vi "Example virtual calibration data generator.vi"(0 "t0_U_cal t0 (m/s)":dbl[](array[numeric])=[0.0018065055399, 0.51984069575, 0.9737, 2.0137147675, 3.036660399, 4.008390834, 5.0589598065, 6.0604802741, 7.0995183408, 8.0765049797, 9.0912586991, 10.081448823, 11.876663392], 1 "t0_Vout_cal t0 (V)":dbl[](array[numeric])=[0.053989069621, 0.62774937057, 0.93949993515, 1.4010595347, 1.714702877, 1.9456688245, 2.1571508535, 2.3284715843, 2.4859547348, 2.6192157707, 2.7474417318, 2.8639088415, 3.0588901316], 3 "time fraction (0...1)":dbl=0.5 min=0.0 max=1.0, 5 "t0_Ta_cal (°C)":dbl[](array[numeric])=[20.994930577, 20.998488576, 21.001202392, 21.00530951, 21.005031565, 21.012907585, 21.024551146, 21.046328275, 21.072132623, 21.111764011, 21.153745433, 21.182721788, 21.208832231], 7 "t1_Vout_cal t0 (V)":dbl[](array[numeric])=[0.045499523163, 0.60666541417, 0.91558652878, 1.3778238233, 1.6925483742, 1.9226294759, 2.1202740657, 2.2916270447, 2.4508691012, 2.5910185776, 2.7221374766, 2.8443260727, 3.0437243334], 9 "t1_U_cal t0 (m/s)":dbl[](array[numeric])=[0.021020600342, 0.51776852003, 0.98012050062, 2.0073197538, 3.0227502489, 3.9782177479, 4.9506397512, 5.9384973419, 6.9603671247, 7.9606730411, 8.9790875099, 10.010118367, 11.844900957], 11 "t1_Ta_cal (°C)":dbl[](array[numeric])=[21.415303275, 21.38340196, 21.380579107, 21.375484666, 21.374167855, 21.37609939, 21.376411452, 21.399550636, 21.436538733, 21.478179347, 21.519214886, 21.536252007, 21.540514259], 12 "Overheat ratio":dbl=1.7, 13 "Gain":dbl=10.0, 14 "Offset (V)":dbl=0.512) -> (4 "t_frac Calibration data":T1={"X cal.[]"=[0.16942387073906073, 0.3571463864829161, 0.4649272045522078, 0.6384095030771939, 0.7632235157537435, 0.8589678745414981, 0.9489717058438498, 1.0240141417905662, 1.0951488178464426, 1.1566490826880553, 1.2166980237427845, 1.2717330176412438, 1.3654642977024674], "Re cal.[]"=[0.0003549732812892601, 0.10214643281768965, 0.19132665434147333, 0.39568017737456973, 0.5966818576867157, 0.7876060754864341, 0.9940059313339666, 1.190731239913453, 1.3947958933586706, 1.5865981769860278, 1.7857758481557438, 1.9801490739357872, 2.332620901742986], "a1[]"=[0.5422442754565113, 0.6848331445720253, 1.0026861494680874, 1.394179926934208, 1.8022568311200722, 2.1436691011118443, 2.4573774667113204, 2.7451146877065913, 2.9937157196852064, 3.217822590174205, 3.424366908750728, 3.6461309534080004], "a2[]"=[-0.7595725454163121, 1.0197881628604482, 0.7741344852897616, 1.927764485021313, 2.4453609640659906, 1.4997878970452068, 2.727694680301364, 1.7175948982636757, 2.4538859657545333, 1.511346978354529, 1.8273792682683536, 2.4393015310094333], "a3[]"=[4.046251683803012, 2.8127827457089394, 1.361156267749989, -1.5651263013416128, -4.612450848415237, 1.7996431474362735, -7.200648409580028, 0.2793016807904881, -6.849691205223936, 2.314255218633881, 2.2697753416122333, -13.012206434266801]}, 10 "t0 Calibration data":T1={"X cal.[]"=[0.16942387073906073, 0.3571463864829161, 0.4649272045522078, 0.6384095030771939, 0.7632235157537435, 0.8589678745414981, 0.9489717058438498, 1.0240141417905662, 1.0951488178464426, 1.1566490826880553, 1.2166980237427845, 1.2717330176412438, 1.3654642977024674], "Re cal.[]"=[0.0003549732812892601, 0.10214643281768965, 0.19132665434147333, 0.39568017737456973, 0.5966818576867157, 0.7876060754864341, 0.9940059313339666, 1.190731239913453, 1.3947958933586706, 1.5865981769860278, 1.7857758481557438, 1.9801490739357872, 2.332620901742986], "a1[]"=[0.5422442754565113, 0.6848331445720253, 1.0026861494680874, 1.394179926934208, 1.8022568311200722, 2.1436691011118443, 2.4573774667113204, 2.7451146877065913, 2.9937157196852064, 3.217822590174205, 3.424366908750728, 3.6461309534080004], "a2[]"=[-0.7595725454163121, 1.0197881628604482, 0.7741344852897616, 1.927764485021313, 2.4453609640659906, 1.4997878970452068, 2.727694680301364, 1.7175948982636757, 2.4538859657545333, 1.511346978354529, 1.8273792682683536, 2.4393015310094333], "a3[]"=[4.046251683803012, 2.8127827457089394, 1.361156267749989, -1.5651263013416128, -4.612450848415237, 1.7996431474362735, -7.200648409580028, 0.2793016807904881, -6.849691205223936, 2.314255218633881, 2.2697753416122333, -13.012206434266801]}, 15 "t1* Calibration data":T1={"X cal.[]"=[0.16942387073906073, 0.3571463864829161, 0.4649272045522078, 0.6384095030771939, 0.7632235157537435, 0.8589678745414981, 0.9489717058438498, 1.0240141417905662, 1.0951488178464426, 1.1566490826880553, 1.2166980237427845, 1.2717330176412438, 1.3654642977024674], "Re cal.[]"=[0.0003549732812892601, 0.10214643281768965, 0.19132665434147333, 0.39568017737456973, 0.5966818576867157, 0.7876060754864341, 0.9940059313339666, 1.190731239913453, 1.3947958933586706, 1.5865981769860278, 1.7857758481557438, 1.9801490739357872, 2.332620901742986], "a1[]"=[0.5422442754565113, 0.6848331445720253, 1.0026861494680874, 1.394179926934208, 1.8022568311200722, 2.1436691011118443, 2.4573774667113204, 2.7451146877065913, 2.9937157196852064, 3.217822590174205, 3.424366908750728, 3.6461309534080004], "a2[]"=[-0.7595725454163121, 1.0197881628604482, 0.7741344852897616, 1.927764485021313, 2.4453609640659906, 1.4997878970452068, 2.727694680301364, 1.7175948982636757, 2.4538859657545333, 1.511346978354529, 1.8273792682683536, 2.4393015310094333], "a3[]"=[4.046251683803012, 2.8127827457089394, 1.361156267749989, -1.5651263013416128, -4.612450848415237, 1.7996431474362735, -7.200648409580028, 0.2793016807904881, -6.849691205223936, 2.314255218633881, 2.2697753416122333, -13.012206434266801]})   [LabVIEW 2022 SP3]
doc: "Example VI for how to pre-process and make use of two sequential calibration datasets to generate a virtual calibration at some fractional time between the two calibration datasets.\nPN 15-OCT-24."
uses:
  Ctls/Calibration data.ctl
panel:
  out "Calibration curves":cluster{dbl[], dbl[]}[](graph)=[{[0.17351078077836318, 0.35960238349240253, 0.46891791081947753, 0.6413681992780179, 0.7657591156025723, 0.8611448971603233, 0.951297198203673, 1.0263676092211313, 1.0969658195169174, 1.1579995632331852, 1.2177718423536772, 1.2728558335390798, 1.3667235881026694], [0.0003549732812892601, 0.10214643281768965, 0.19132665434147333, 0.39568017737456973, 0.5966818576867157, 0.7876060754864341, 0.9940059313339666, 1.190731239913453, 1.3947958933586706, 1.5865981769860278, 1.7857758481557438, 1.9801490739357872, 2.332620901742986]}, {[0.16533696069975826, 0.3546903894734296, 0.4609364982849381, 0.6354508068763699, 0.7606879159049147, 0.856790851922673, 0.9466462134840266, 1.0216606743600007, 1.0933318161759675, 1.1552986021429255, 1.2156242051318917, 1.2706102017434078, 1.3642050073022656], [0.0003549732812892601, 0.10214643281768965, 0.19132665434147333, 0.39568017737456973, 0.5966818576867157, 0.7876060754864341, 0.9940059313339666, 1.190731239913453, 1.3947958933586706, 1.5865981769860278, 1.7857758481557438, 1.9801490739357872, 2.332620901742986]}, {[0.16942387073906073, 0.3571463864829161, 0.4649272045522078, 0.6384095030771939, 0.7632235157537435, 0.8589678745414981, 0.9489717058438498, 1.0240141417905662, 1.0951488178464426, 1.1566490826880553, 1.2166980237427845, 1.2717330176412438, 1.3654642977024674], [0.0003549732812892601, 0.10214643281768965, 0.19132665434147333, 0.39568017737456973, 0.5966818576867157, 0.7876060754864341, 0.9940059313339666, 1.190731239913453, 1.3947958933586706, 1.5865981769860278, 1.7857758481557438, 1.9801490739357872, 2.332620901742986]}]
  # "Note: t0 and t1 arrays must have the same length."
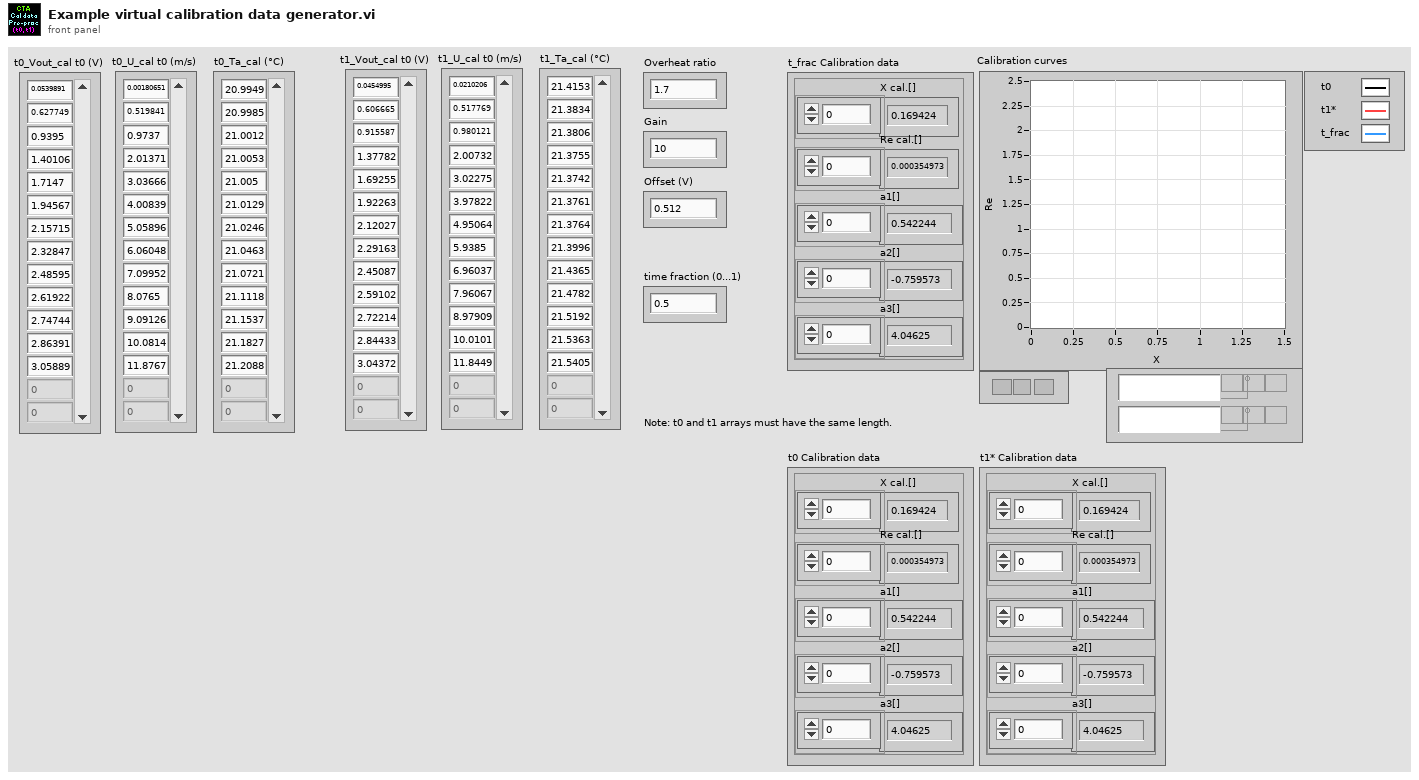
[diagram p1: front panel]
types:
  T1 = typedef "Calibration data.ctl" = cluster{"X cal.[]":dbl[], "Re cal.[]":dbl[], "a1[]":dbl[], "a2[]":dbl[], "a3[]":dbl[]}
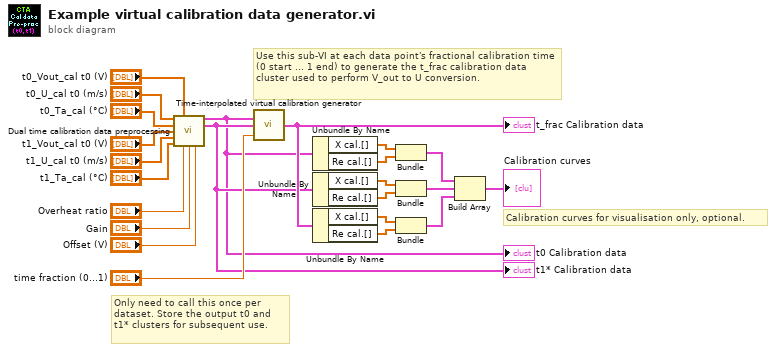
[diagram p0: block diagram]
diagram:
  # "Calibration curves for visualisation only, optional."
  # "Use this sub-VI at each data point's fractional calibration time (0 start ... 1 end) to generate the t_frac calibration data cluster used to perform V_out to U conversion."
  # "Only need to call this once per dataset. Store the output t0 and t1* clusters for subsequent use."
  n1 = call "Dual time calibration data preprocessing.vi"("t0_U_cal t0 (m/s)"="t0_U_cal t0 (m/s)", "t0_Vout_cal t0 (V)"="t0_Vout_cal t0 (V)", "t0_Ta_cal (°C)"="t0_Ta_cal (°C)", "t1_Vout_cal t0 (V)"="t1_Vout_cal t0 (V)", "t1_U_cal t0 (m/s)"="t1_U_cal t0 (m/s)", "t1_Ta_cal (°C)"="t1_Ta_cal (°C)", "Overheat ratio"="Overheat ratio", "Gain"="Gain", "Offset (V)"="Offset (V)") -> ("t0 Calibration data"=w1:T1, "t1* Calibration data"=w2:T1)  [unwired: 5 in]
  "t0 Calibration data" <- w1
  "t1* Calibration data" <- w2
  n2 = call "Time-interpolated virtual calibration generator.vi"("time fraction (0...1)"="time fraction (0...1)", "t1* Calibration data"=w2, "t0 Calibration data"=w1) -> ("t_frac Calibration data"=w3:T1)
  "t_frac Calibration data" <- w3
  n3 = Unbundle By Name(w1) -> ("X cal.[]"=w9:dbl[], "Re cal.[]"=w6:dbl[])
  n4 = Unbundle By Name(w2) -> ("X cal.[]"=w8:dbl[], "Re cal.[]"=w5:dbl[])
  n5 = Unbundle By Name(w3) -> ("X cal.[]"=w7:dbl[], "Re cal.[]"=w4:dbl[])
  n6 = Bundle("X cal.[]"=w9, "Re cal.[]"=w6) -> (w11:cluster{"X cal.[]":dbl[], "Re cal.[]":dbl[]})  [unwired: 1 in]
  n7 = Bundle("X cal.[]"=w8, "Re cal.[]"=w5) -> (w12:cluster{"X cal.[]":dbl[], "Re cal.[]":dbl[]})  [unwired: 1 in]
  n8 = Bundle("X cal.[]"=w7, "Re cal.[]"=w4) -> (w13:cluster{"X cal.[]":dbl[], "Re cal.[]":dbl[]})  [unwired: 1 in]
  n9 = Build Array(w11, w12, w13) -> (→"Calibration curves":cluster{"X cal.[]":dbl[], "Re cal.[]":dbl[]}[])
